vi "Initialize HW.vi"(8 "error in (no error)":errorcluster, 11 "Simulated Switch in":refnum<class "Simulated Switch.lvclass">) -> (0 "error out":errorcluster, 3 "Simulated Switch out":refnum<class "Simulated Switch.lvclass">)   [LabVIEW 2020, in "Simulated Switch.lvclass"]
uses:
  Simulated Switch.lvclass
  Switch.lvclass
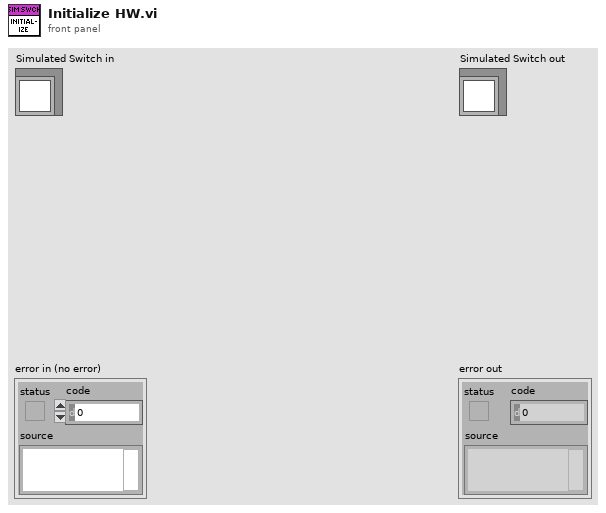
[diagram p1: front panel]
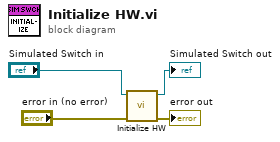
[diagram p0: block diagram]
diagram:
  n1 = call-parent "Initialize HW.vi"("error in (no error)"="error in (no error)", "Switch in"="Simulated Switch in") -> ("error out"=→"error out":errorcluster, "Switch out"=→"Simulated Switch out":refnum<class "Simulated Switch.lvclass">)  [unwired: 8 in]
